vi "PH_Beckhoff_Application.panel.vi"(0 "object ref":refnum<vi>, 5 "error in (no error)":errorcluster) -> (19 "error out":errorcluster)   [LabVIEW 2014, in "PH_Beckhoff_Application.lvlib"]
doc: "This a GUI.\n\nLicense Agreement for this software:\n\nCopyright (C)\nGesellschaft für Schwerionenforschung, GSI\nPlanckstr. 1\n64291 Darmstadt\nGermany\n\nContact: D.Beck@gsi.de \n\nThis program is free software; you can redistribute it and/or modify it under the terms of the GNU General Public License as published by the Free Software Foundation; either version 2 of the license, or (at your option) any later version.\n\nThis program is distributed in the hope that it will be useful, but WITHOUT ANYW ARRANTY; without even the implied warranty of MERCHANTABILITY or FITNESS FOR A PARTICULAR PURPOSE. See the GNU General License for more details (http://www.gnu.org).\n\nGesellschaft für Schwerionenforschung, GSI\nPlanckstr. 1, 64291 Darmstadt, Germany\nFor all questions and ideas contact: M.Richter@gsi.de, H.Brand@gsi.de or D.Beck@gsi.de.\nLast update: 18-DEC-2002"
uses:
  PH_Beckhoff_Application.lvlib
  PH_Beckhoff/PH_Beckhoff.Connectivity.ctl
  PH_Beckhoff/PH_Beckhoff.Values.ctl
  PH_Beckhoff/PH_Beckhoff.Sonderklemmen Inputs.ctl
  PH_Beckhoff/PH_Beckhoff.Analog Inputs.ctl
  PH_Beckhoff/PH_Beckhoff.Scaling Type.ctl
  PH_Beckhoff/PH_Beckhoff.Analog Outputs.ctl
  PH_Beckhoff/PH_Beckhoff.Digital Inputs.ctl
  PH_Beckhoff/PH_Beckhoff.Digital Outputs.ctl
  PH_Beckhoff/PH_Beckhoff.ADS Error.ctl
  PH_Beckhoff_Application.Beckhoff Type.ctl
  PH_Beckhoff/PH_Beckhoff.GUI Refs.ctl
  CS_Core/CSObj/CSObj.lvlib
  PH_Basics/PH_Common/PH_Common.lvlib
  PH_Beckhoff/PH_Beckhoff.lvlib
  CS_Core/CSSystem/CSSystemLib/CSSystemLib.lvlib
  PH_Basics/PH_Class/PH_Class.lvlib
panel:
  out "Beckhoff Type":T1
  out "configured?":bool
  out "ADS Error":T2
  in  "Show Info":bool
  out "Values":T3
  out "Prdc Int [ms]":i32
  out "Connection":T10
  out "IP":string
  in  "Delete":bool
  in  "Exit":bool
  # "PCS"
  # "3.40"
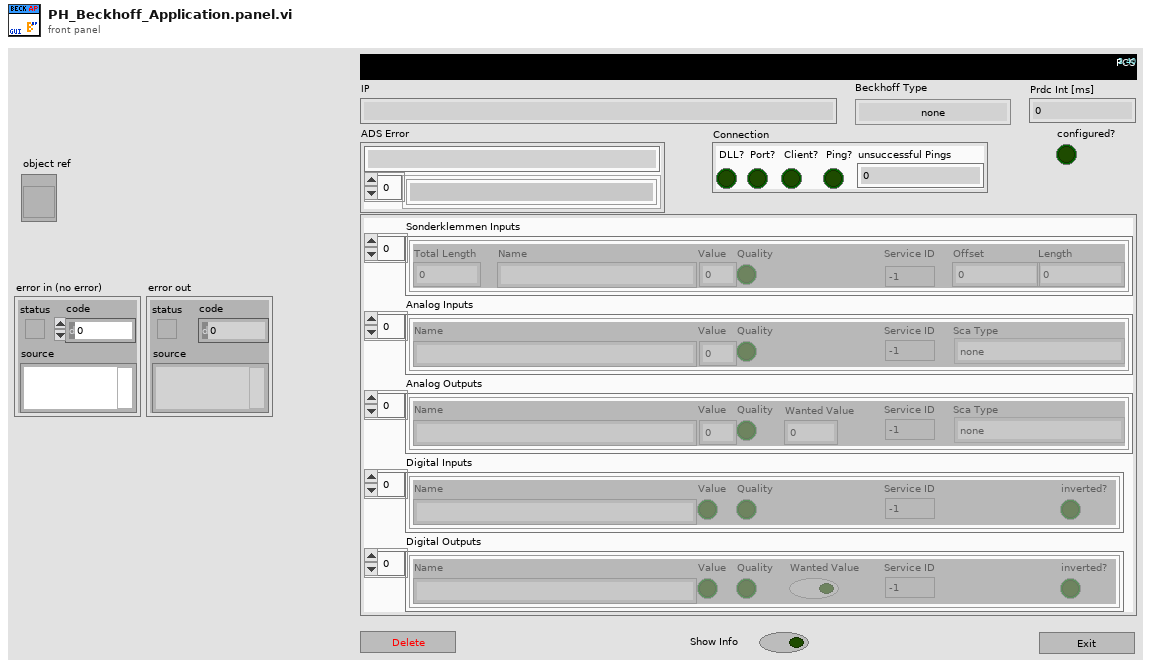
[diagram p1: front panel]
types:
  T1 = typedef "PH_Beckhoff_Application.lvlib/PH_Beckhoff_Application.Beckhoff Type.ctl" = enum16{"none", "PILS internal", "PILS external", "Timing", "MA 01"}
  T2 = typedef "PH_Beckhoff.lvlib/PH_Beckhoff.ADS Error.ctl" = cluster{"Latest Error":string, "Error List":string[]}
  T3 = typedef "PH_Beckhoff.lvlib/PH_Beckhoff.Values.ctl" = cluster{"Sonderklemmen Inputs":T4, "Analog Inputs":T5, "Analog Outputs":T7, "Digital Inputs":T8, "Digital Outputs":T9}
  T4 = typedef "PH_Beckhoff.lvlib/PH_Beckhoff.Sonderklemmen Inputs.ctl" = cluster{"Total Length":u32, "Name":string, "Value":u64, "Quality":bool, "Service ID":i32, "Offset":u32, "Length":u32}[]
  T5 = typedef "PH_Beckhoff.lvlib/PH_Beckhoff.Analog Inputs.ctl" = cluster{"Name":string, "Value":u32, "Quality":bool, "Service ID":i32, "Sca Type":T6}[]
  T6 = typedef "PH_Beckhoff.lvlib/PH_Beckhoff.Scaling Type.ctl" = enum16{"none", "0 ... 15 Bit -> 0 ... 5", "0 ... 15 Bit -> 0 ... 10", "0 ... 15 Bit -> 0 ... 25", "0 ... 15 Bit -> 4 ... 20", "0 ... 15 Bit -> 0 ... 1", "0 ... 15 Bit -> 0 ... 20000", "0 ... 15 Bit -> 0 ... 24000"}
  T7 = typedef "PH_Beckhoff.lvlib/PH_Beckhoff.Analog Outputs.ctl" = cluster{"Name":string, "Value":u32, "Quality":bool, "Wanted Value":u32, "Service ID":i32, "Sca Type":T6}[]
  T8 = typedef "PH_Beckhoff.lvlib/PH_Beckhoff.Digital Inputs.ctl" = cluster{"Name":string, "Value":bool, "Quality":bool, "Service ID":i32, "inverted?":bool}[]
  T9 = typedef "PH_Beckhoff.lvlib/PH_Beckhoff.Digital Outputs.ctl" = cluster{"Name":string, "Value":bool, "Quality":bool, "Wanted Value":bool, "Service ID":i32, "inverted?":bool}[]
  T10 = typedef "PH_Beckhoff.lvlib/PH_Beckhoff.Connectivity.ctl" = cluster{"DLL?":bool, "Port?":bool, "Client?":bool, "Ping?":bool, "unsuccessful Pings":u32}
  T11 = typedef "PH_Beckhoff.lvlib/PH_Beckhoff.GUI Refs.ctl" = cluster{"ADS Error":refnum<vi>, "Values":refnum<vi>, "configured?":refnum<vi>, "Connection":refnum<vi>, "IP":refnum<vi>, "Prdc Int [ms]":refnum<vi>}
  T12 = typedef "PH_Beckhoff.lvlib/PH_Beckhoff.i attribute.ctl" = cluster{"GUI Refs":T11, "operation?":bool, "Default Prdc Interval":i32, "Connection":T10, "AMS Net ID":T13, "Klemmencluster: # of":T14, "Values":T3, "IP":string, "Description":string, "configured?":bool, "Change Manager":cluster{"Detemination wanted?":bool, "Values changed at":cluster{"Sonderklemmen Inputs":i32[], "Analog Inputs":i32[], "Analog Outputs":i32[], "Digital Inputs":i32[], "Digital Outputs":i32[]}}, "Difference to handle an analog input as change":u32}
  T13 = typedef "Beckhoff - Driver np.lvlib/Beckhoff Access.ctl" = cluster{"DLL path":path, "AMS Net ID":cluster{"1st # of IP":u8, "2nd # of IP":u8, "3rd # of IP":u8, "4th # of IP":u8, "In Port":u8, "Out Port":u8}}
  T14 = typedef "Beckhoff - Driver np.lvlib/Klemmendeclarer.ctl" = cluster{"Offset due to Sonderklemms":u32, "analog Inputs":u32, "analog Outputs":u32, "digital Input Bits":u32, "digital Output Bits":u32}
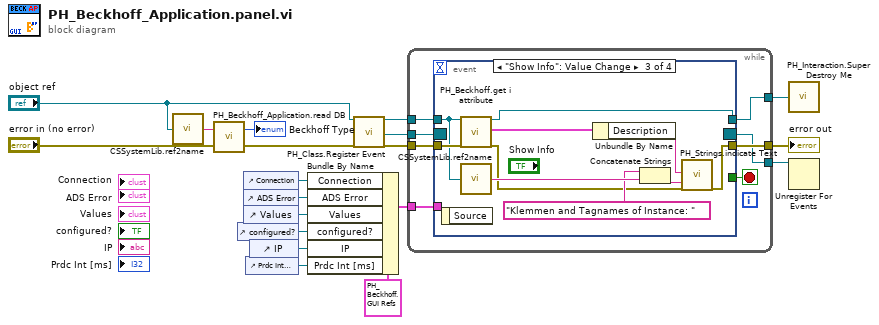
[diagram p0: block diagram]
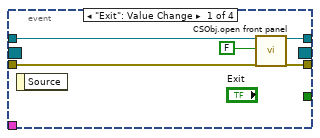
[diagram p2: hidden frame]
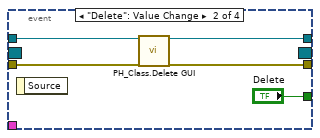
[diagram p3: hidden frame]
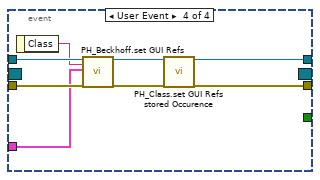
[diagram p4: hidden frame]
diagram:
  n1 = call "CSSystemLib.ref2name.vi"("obj refnum"="object ref") -> ("name"=w1:string)
  n2 = call "PH_Beckhoff_Application.read DB.vi"("error in"="error in (no error)", "Instance Name"=w1) -> ("error out"=w10:errorcluster, "Beckhoff Type"=→"Beckhoff Type":T1)
  n3 = control-ref of="configured?"() -> (w13:refnum<vi>)
  n4 = control-ref of="Connection"() -> (w17:refnum<vi>)
  n5 = control-ref of="ADS Error"() -> (w15:refnum<vi>)
  n6 = control-ref of="Values"() -> (w16:refnum<vi>)
  n7 = control-ref of="Prdc Int [ms]"() -> (w3:refnum<vi>)
  n8 = control-ref of="IP"() -> (w4:refnum<vi>)
  n9 = Bundle By Name(cluster=T11 {"ADS Error"=refnum, "Values"=refnum, "configured?"=refnum, "Connection"=refnum, "IP"=refnum, "Prdc Int [ms]"=refnum} ("GUI Refs"), "Connection"=w17, "ADS Error"=w15, "Values"=w16, "configured?"=w13, "IP"=w4, "Prdc Int [ms]"=w3) -> (w6:T11)
  n10 = call "PH_Class.Register Event.vi"("i ref in"="object ref", "error in (no error)"=w10) -> ("i ref out"=w11:refnum<vi>, "Event Registration Refnum"=w8:refnum<event-registration>, "error out"=w9:errorcluster)  [unwired: 15 in]
  n11 = while {
    tunnel: w11 -> [w24]
    tunnel: [w23] -> w19
    tunnel: w9 -> [w26]
    tunnel: [w25] -> w18
    tunnel: w8 -> [w22]
    tunnel: [w21] -> w7
    tunnel: w6 -> [w20]
    stop <- w27 stop-if-true
    n12 = event shown="[2] \"Show Info\": Value Change" {
      selector: w22 -> [_ _ _ _]
      dyn-events: [_ _ _ _] -> w21
      timeout: _ -> [_ _ _ _]
      tunnel: [_ "Delete" _ _] -> w27
      tunnel: w24 -> [w29 w34 w38 w55]
      tunnel: w26 -> [w32 w36 w41 w54]
      tunnel: [w31 w35 w39 w50] -> w25
      tunnel: [w28 w33 w40 w48] -> w23
      tunnel: w20 -> [_ _ _ w51]
      event "Exit": Value Change {
        n13 = event-data() -> ()  [unwired: 1 in, 1 out]
        n14 = call "CSObj.open front panel.vi"("i ref in"=w29, "frontPanelOpen"=FALSE ("front panel open"), "error in (no error)"=w32) -> ("i ref out"=w28:refnum<vi>, "error out"=w31:errorcluster)  [unwired: 15 in]
      }
      event "Delete": Value Change {
        n15 = event-data() -> ()  [unwired: 1 in, 1 out]
        n16 = call "PH_Class.Delete GUI.vi"("VI in"=w34, "error in (no error)"=w36) -> ("VI out"=w33:refnum<vi>, "error out"=w35:errorcluster)  [unwired: 16 in]
      }
      event "Show Info": Value Change {
        n17 = event-data() -> ()  [unwired: 1 in, 1 out]
        n18 = call "PH_Beckhoff.get i attribute.vi"("i ref in"=w38, "error in (no error)"=w41) -> ("i ref out"=w40:refnum<vi>, "i attribute"=w43:T12, "error out"=w42:errorcluster)  [unwired: 15 in]
        n19 = call "CSSystemLib.ref2name.vi"("obj refnum"=w38) -> ("name"=w47:string)
        n20 = Unbundle By Name(w43) -> ("Description"=w44:string)
        n21 = Concatenate Strings("Klemmen and Tagnames of Instance: " ("Caption.Text"), w47) -> (w46:string)
        n22 = call "PH_Strings.indicate Text.vi"("String to show"=w44, "Caption.Text"=w46, "error in (no error)"=w42) -> ("error out"=w39:errorcluster)  [unwired: 16 in]
      }
      event User Event {
        n23 = event-data() -> ("Class"=w52:string)  [unwired: 1 in]
        n24 = call "PH_Beckhoff.set GUI Refs.vi"("i ref in"=w55, "Class"=w52, "GUI Refs"=w51, "error in"=w54) -> ("i ref out"=w49:refnum<vi>, "error out"=w53:errorcluster)  [unwired: 14 in]
        n25 = call "PH_Class.set GUI Refs stored Occurence.vi"("i ref in"=w49, "error in (no error)"=w53) -> ("i ref out"=w48:refnum<vi>, "error out"=w50:errorcluster)  [unwired: 16 in]
      }
    }
  }
  "error out" <- w18
  n26 = call "PH_Interaction.Super Destroy Me.vi"("i ref out"=w19) -> ()
  n27 = Unregister For Events(event registration refnum=w7) -> ()  [unwired: 1 in, 1 out]
